vi "ParseText.vi"(8 "error in (no error)":errorcluster, 10 "textFragmentDefault in":T1, 11 "text in":string) -> (0 "error out":errorcluster, 2 "textFragments out":T1[](array[typedef]), 3 "text out":string)   [LabVIEW 2010, in "StyledText.lvlib"]
doc: "Parses the given styled text. Returns the plain text as a single string and the text fragments with the style information.\n\n<b ></b > Bold\n<i></i> Italic\n<s></s> or <strike></strike> Strikeout\n<u></u> Underline\n<font></font> Font attributes. Currently supported are face, color and size. Colors must be specified in HTML hexadecimal format.\nExample: <font face=\"Courier\" color=\"#FF0000\" size=\"18\">Blabla</font>\n\n<b>Note that the input text must be well-formed XML content, i.e. every tag must be properly closed and text must be properly escaped.</b>\n\nCopyright (c) 2018, Martin Weiss\nAll rights reserved.\n\nRedistribution and use in source and binary forms, with or without modification, are permitted provided that the following conditions are met:\n\n1. Redistributions of source code must retain the above copyright notice, this list of conditions and the following disclaimer.\n\n2. Redistributions in binary form must reproduce the above copyright notice, this list of conditions and the following disclaimer in the documentation and/or other materials provided with the distribution.\n\nTHIS SOFTWARE IS PROVIDED BY THE COPYRIGHT HOLDERS AND CONTRIBUTORS \"AS IS\" AND ANY EXPRESS OR IMPLIED WARRANTIES, INCLUDING, BUT NOT LIMITED TO, THE IMPLIED WARRANTIES OF MERCHANTABILITY AND FITNESS FOR A PARTICULAR PURPOSE ARE DISCLAIMED. IN NO EVENT SHALL THE COPYRIGHT HOLDER OR CONTRIBUTORS BE LIABLE FOR ANY DIRECT, INDIRECT, INCIDENTAL, SPECIAL, EXEMPLARY, OR CONSEQUENTIAL DAMAGES (INCLUDING, BUT NOT LIMITED TO, PROCUREMENT OF SUBSTITUTE GOODS OR SERVICES; LOSS OF USE, DATA, OR PROFITS; OR BUSINESS INTERRUPTION) HOWEVER CAUSED AND ON ANY THEORY OF LIABILITY, WHETHER IN CONTRACT, STRICT LIABILITY, OR TORT (INCLUDING NEGLIGENCE OR OTHERWISE) ARISING IN ANY WAY OUT OF THE USE OF THIS SOFTWARE, EVEN IF ADVISED OF THE POSSIBILITY OF SUCH DAMAGE."
uses:
  StyledText.lvlib
  TextFragment.ctl
  <vilib>/Utility/miscctls.llb/LVSelectionTypeDef.ctl
  <vilib>/Utility/miscctls.llb/LVFontTypeDef.ctl
  <vilib>/xml/Load XML String.vi
  <vilib>/xml/Close Reference(Node).vi
  <vilib>/xml/NI_XML.lvlib
  Program Files (x86)/National Instruments/LabVIEW 2010/resource/objmgr/DOMUserDefRef.rc
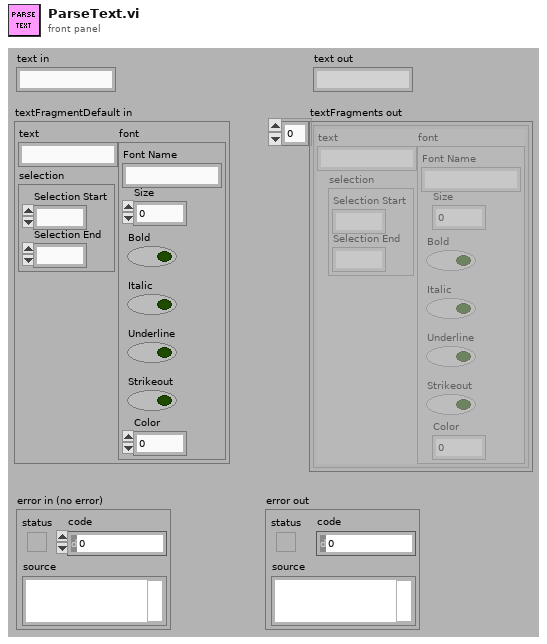
[diagram p1: front panel]
types:
  T1 = typedef "StyledText.lvlib/TextFragment.ctl" = cluster{"text":string, "selection":T2, "font":T3}
  T2 = typedef "LVSelectionTypeDef.ctl" = cluster{"Selection Start":u32, "Selection End":u32}
  T3 = typedef "LVFontTypeDef.ctl" = cluster{"Font Name":string, "Size":u16, "Bold":bool, "Italic":bool, "Underline":bool, "Strikeout":bool, "Color":u32}
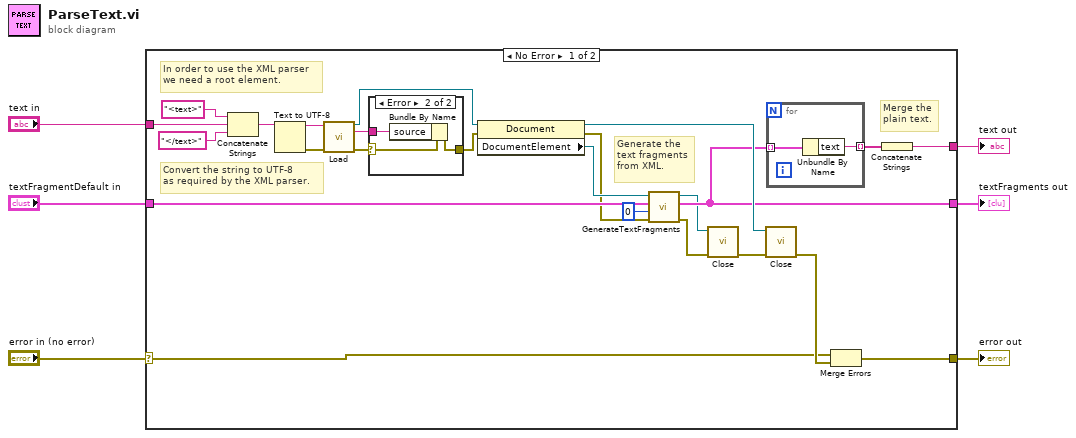
[diagram p0: block diagram]
diagram:
  n1 = case shown="No Error" "error in (no error)" {
    selector: "error in (no error)" -> [w19 w37]
    tunnel: [w11 w37] -> w5
    tunnel: [w21 _] -> w4
    tunnel: "text in" -> [w20 _]
    tunnel: "textFragmentDefault in" -> [w18 _]
    tunnel: [w15 _] -> w1
    frame No Error {
      # "Generate the\ntext fragments\nfrom XML."
      # "Merge the\nplain text."
      # "Convert the string to UTF-8\nas required by the XML parser."
      # "In order to use the XML parser\nwe need a root element."
      n2 = Concatenate Strings("<text>" ("string"), w20, "</text>" ("string")) -> (w26:string)
      n3 = Text to UTF-8(11:w26) -> (0:w29:errorcluster, 3:w27:string)  [unwired: 1 in]
      n4 = call-poly <vilib>:"Load.vi"("XML string"=w27, "error in (no error)"=w29) -> ("DOM document out"=w28:refnum<k20>, "parse errors"=w12:string, "error out"=w14:errorcluster)  [unwired: 11 in]
      n5 = case shown="Error" w14 {
        selector: w14 -> [w33 w36]
        tunnel: [w33 w35] -> w13
        tunnel: w12 -> [_ w34]
        frame No Error {
        }
        frame Error {
          n6 = Bundle By Name(cluster=w36, "source"=w34) -> (w35:errorcluster)
        }
      }
      n7 = property class="Document"(reference=w28, error in=w13) -> (reference out=w25:refnum<k20>, error out=w9:errorcluster, "DocumentElement"=w10:refnum<k20>)
      n8 = call "GenerateTextFragments.vi"("error in (no error)"=w9, "textPosition in"=u32 0, "textFragment in"=w18, "xmlelement in"=w10) -> ("error out"=w8:errorcluster, "textFragments out"=w21:T1[], "xmlelement out"=w7:refnum<k20>)  [unwired: 4 in, 1 out]
      n9 = call-poly <vilib>:"Close.vi"("error in (no error)"=w8, "node"=w7) -> ("error out"=w24:errorcluster)  [unwired: 7 in]
      n10 = call-poly <vilib>:"Close.vi"("error in (no error)"=w24, "node"=w25) -> ("error out"=w30:errorcluster)  [unwired: 7 in]
      n11 = for {
        tunnel: w21 -> [w32] mode=indexing
        tunnel: [w31] -> w16 mode=indexing
        n12 = Unbundle By Name(w32) -> ("text"=w31:string)
      }
      n13 = Merge Errors(w19, w30) -> (w11:errorcluster)
      n14 = Concatenate Strings(w16) -> (w15:string)
    }
    frame Error {
    }
  }
  "error out" <- w5
  "textFragments out" <- w4
  "text out" <- w1
